vi "SDCP SMF Receiver and Transmitter - Tx Base.vi"(1 "error in (no error)":errorcluster) -> (0 "error out":errorcluster)   [LabVIEW 2020]
uses:
  Typedefs/SDCP - Serial Port Control - Commands.ctl
  Typedefs/SDCP SMF logger - SMF with timestamp.ctl
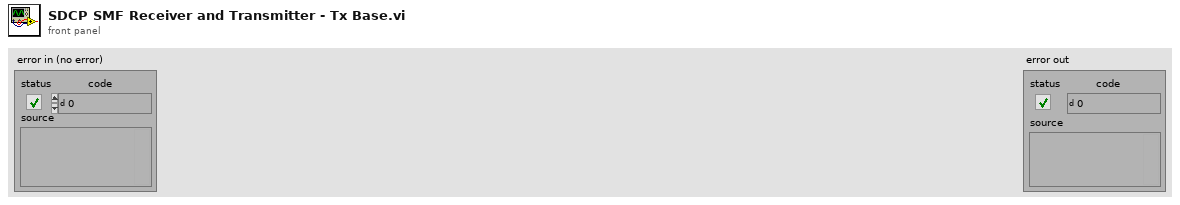
[diagram p1: front panel]
types:
  T1 = typedef "SDCP - Serial Port Control - Commands.ctl" = enum16{"Open", "Read", "Write", "Get instance", "Close"}
  T2 = typedef "SDCP SMF Receiver and Transmitter - Notifier and Queues.ctl" = cluster{"Trace Queue":refnum<queue>, "Tx - Log Table Queue":refnum<queue>, "Tx - User Queue":refnum<queue>, "Rx - Log Table Queue":refnum<queue>, "Rx - User Queue":refnum<queue>, "Log status Notifier":refnum<notifier>, "Plot Queue":refnum<queue>}
  T3 = typedef "SDCP SMF logger - SMF with timestamp.ctl" = cluster{"Bytes":u8[], "Checksum":bool, "Time (ms)":u32, "Tx/Rx":string}
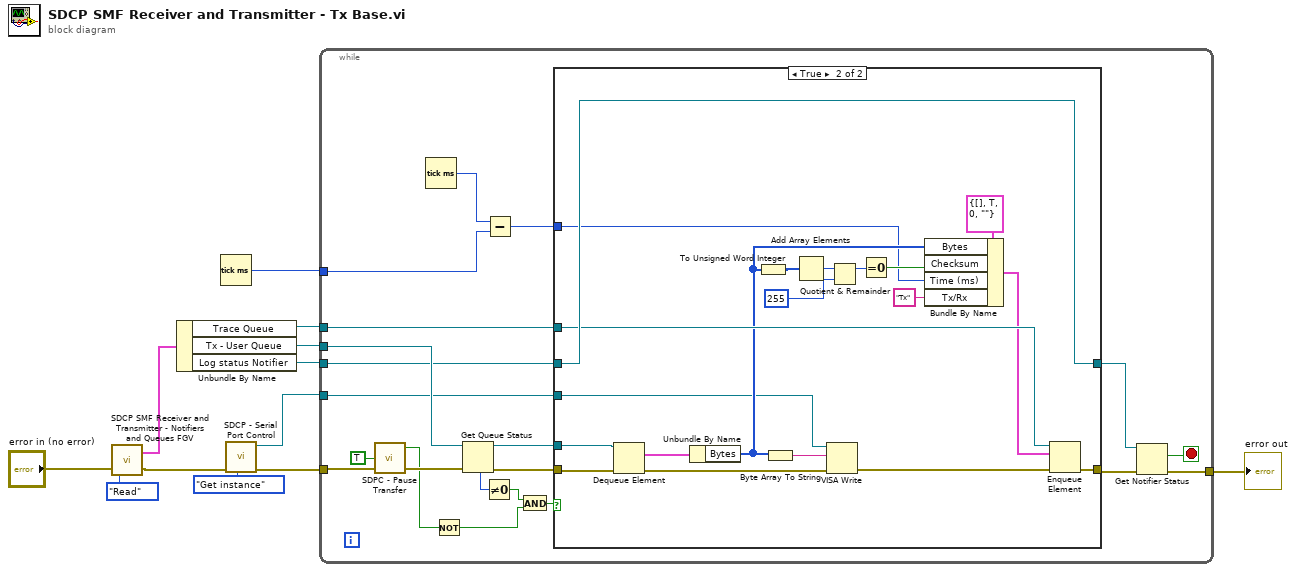
[diagram p0: block diagram]
diagram:
  n1 = call "SDCP SMF Receiver and Transmitter - Notifiers and Queues FGV.vi"("error in (no error)"="error in (no error)", "Command"=enum16{"Initialize", "Read", "Deinitialize"}."Read") -> ("error out"=w4:errorcluster, "Output"=w10:T2)
  n2 = Unbundle By Name(w10) -> ("Trace Queue"=w9:refnum<queue>, "Tx - User Queue"=w7:refnum<queue>, "Log status Notifier"=w6:refnum<notifier>)
  n3 = Tick Count (ms)() -> (millisecond timer value=w8:u32)
  n4 = call "SDCP - Serial Port Control.vi"("Command"=SDCP_-_Serial_Port_Control_-_Commands."Get instance", "error in (no error)"=w4) -> ("error out"=w3:errorcluster, "VISA out"=w1:refnum<visa-resource-name>)  [unwired: 6 in, 2 out]
  n5 = while {
    tunnel: w3 -> [w19]
    tunnel: w9 -> [w21]
    tunnel: w8 -> [w29]
    tunnel: w7 -> [w33]
    tunnel: w6 -> [w27]
    tunnel: [w22] -> w5
    tunnel: w1 -> [w20]
    stop <- w24 stop-if-true
    n6 = call "SDPC - Pause Transfer.vi"("error in (no error)"=w19, "RD/nWR"=TRUE) -> ("error out"=w18:errorcluster, "Transfer paused"=w16:bool)  [unwired: 2 in]
    n7 = Tick Count (ms)() -> (millisecond timer value=w30:u32)
    n8 = Not(x=w16) -> (.not. x?=w13:bool)
    n9 = Get Queue Status(queue=w33, error in (no error)=w18) -> (queue out=w23:refnum<queue>, error out=w31:errorcluster, # elements in queue=w32:i32)  [unwired: 1 in, 5 out]
    n10 = Not Equal To 0?(x=w32) -> (x != 0?=w14:bool)
    n11 = Subtract(x=w30, y=w29) -> (x-y=w28:u32)
    n12 = And(x=w14, y=w13) -> (x .and. y?=w15:bool)
    n13 = case shown="True" w15 {
      tunnel: w31 -> [w35 w54]
      tunnel: w28 -> [_ w39]
      tunnel: w27 -> [w34 w55]
      tunnel: [w35 w48] -> w26
      tunnel: [w34 w55] -> w25
      tunnel: w23 -> [_ w53]
      tunnel: w21 -> [_ w47]
      tunnel: w20 -> [_ w36]
      frame False {
      }
      frame True {
        n14 = Dequeue Element(queue=w53, error in (no error)=w54) -> (element=w52:T3, error out=w51:errorcluster)  [unwired: 1 in, 2 out]
        n15 = Unbundle By Name(w52) -> ("Bytes"=w45:u8[])
        n16 = To Unsigned Word Integer(number=w45) -> (unsigned 16bit integer=w44:u16[])
        n17 = Byte Array To String(unsigned byte array=w45) -> (string=w50:string)
        n18 = Add Array Elements(numeric array=w44) -> (sum=w43:u16)
        n19 = VISA Write(VISA resource name=w36, write buffer=w50, error in (no error)=w51) -> (error out=w49:errorcluster)  [unwired: 2 out]
        n20 = Quotient & Remainder(x=w43, y=u16 255) -> (x-y*floor(x/y)=w41:u16)  [unwired: 1 out]
        n21 = Equal To 0?(x=w41) -> (x = 0?=w40:bool)
        n22 = Bundle By Name(cluster=T3 {"Bytes"=[], "Checksum"=TRUE, "Time (ms)"=0, "Tx/Rx"=""} ("element"), "Bytes"=w45, "Checksum"=w40, "Time (ms)"=w39, "Tx/Rx"="Tx") -> (w37:T3)
        n23 = Enqueue Element(queue=w47, element=w37, error in (no error)=w49) -> (error out=w48:errorcluster)  [unwired: 1 in, 2 out]
      }
    }
    n24 = Get Notifier Status(notifier=w25, error in (no error)=w26) -> (current notification=w24:bool, error out=w22:errorcluster)  [unwired: 3 out]
  }
  "error out" <- w5
